vi "swap slashes.vi"(11 "in":string) -> (3 "out":string)   [LabVIEW 2018]
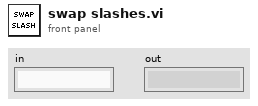
[diagram p1: front panel]
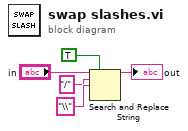
[diagram p0: block diagram]
diagram:
  n1 = Search and Replace String(replace all?=TRUE ("replace all? (F)"), input string="in", search string="/", replace string="\\" ("replace string (\"\")")) -> (result string=→"out":string)  [unwired: 4 in, 3 out]
